vi "marshalling.vi"(8 "error in (no error)":errorcluster, 10 "Variant":variant, 11 "Serializer in":refnum<class "Serializer.openg-ini.lvclass">) -> (0 "error out":errorcluster, 2 "String":string, 3 "Serializer":refnum<class "Serializer.openg-ini.lvclass">)   [LabVIEW 2019, in "OpenSerializer.OpenG-ini.lvlib" / "Serializer.openg-ini.lvclass"]
uses:
  Serializer.openg-ini.lvclass
  Serializer.openg-ini.lvclass/Serializer.openg-ini.ctl
  <vilib>/Utility/config.llb/NI_LVConfig.lvlib
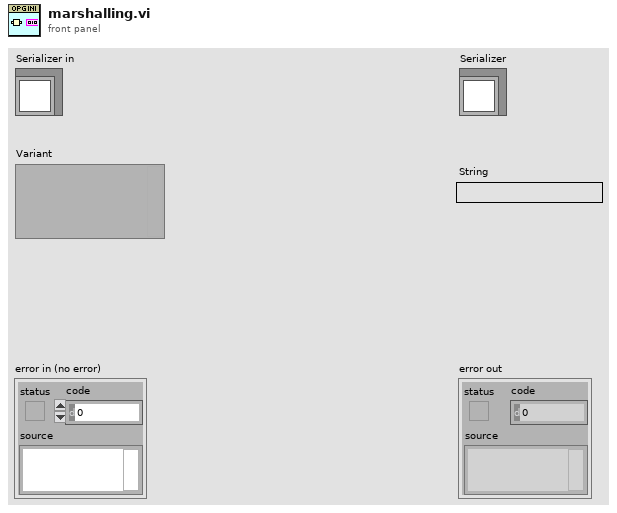
[diagram p1: front panel]
types:
  T1 = enum16{"open", "replace", "create", "open or create", "replace or create", "replace or create with confirmation"}
  T2 = typedef "NI_LVConfig.lvlib/Config Data RefNum.ctl" = refnum<k1>
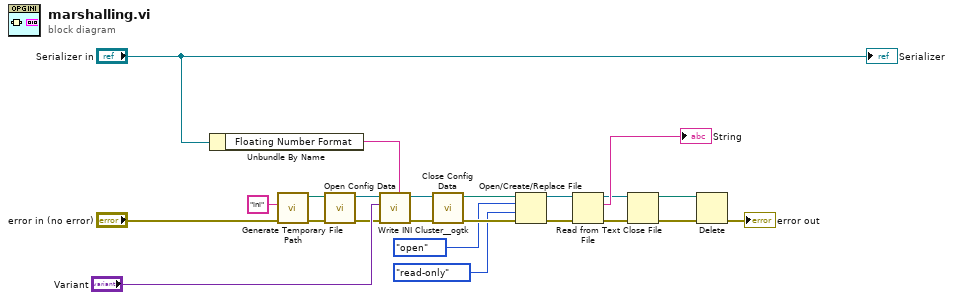
[diagram p0: block diagram]
diagram:
  n1 = Unbundle By Name("Serializer in") -> ("Floating Number Format"=w1:string)
  n2 = call <vilib>:"Generate Temporary File Path.vi"("error in (no error)"="error in (no error)", "Temporary File Extension (tmp)"="ini") -> ("error out"=w21:errorcluster, "Unique Temporary File Path"=w3:path)  [unwired: 8 in]
  n3 = call <vilib>:"Open Config Data.vi"("error in (no error)"=w21, "configuration file path"=w3) -> ("error out"=w20:errorcluster, "refnum"=w19:T2)  [unwired: 7 in, 1 out]
  n4 = call <userlib>:"Write INI Cluster__ogtk.vi"("float number format (optional)"=w1, "error in (no error)"=w20, "INI Fomatted Cluster"="Variant", "refnum"=w19) -> ("error out"=w18:errorcluster, "dup refnum"=w17:T2)  [unwired: 6 in]
  n5 = call <vilib>:"Close Config Data.vi"("error in (no error)"=w18, "refnum"=w17) -> ("error out"=w16:errorcluster, "file path"=w15:path)  [unwired: 8 in]
  n6 = Open/Create/Replace File(file path (use dialog)=w15, error in=w16, operation (0:open)=T1."open", access (0:read/write)=enum16{"read/write", "read-only", "write-only"}."read-only") -> (refnum out=w12:refnum<file>, error out=w11:errorcluster)  [unwired: 2 in, 1 out]
  n7 = Read from Text File(file (use dialog)=w12, error in=w11) -> (refnum out=w8:refnum<file>, text=→"String":string, error out=w9:errorcluster)  [unwired: 2 in, 1 out]
  n8 = Close File(refnum=w8, error in=w9) -> (path=w5:path, error out=w7:errorcluster)
  n9 = Delete(path (use dialog)=w5, error in=w7) -> (error out=→"error out":errorcluster)  [unwired: 3 in, 2 out]
  "Serializer" <- "Serializer in"
